vi "Convert_Meters_to_Inches.vi"   [LabVIEW 2011]
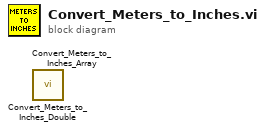
[diagram p0: block diagram]
diagram:
  n1 = call "Convert_Meters_to_Inches_Double.vi"() -> ()  [unwired: 5 in, 1 out]
  n2 = call "Convert_Meters_to_Inches_Array.vi"() -> ()  [unwired: 5 in, 1 out]
